vi "SendMessage.vi"(0 "reference in":refnum<class "Colleague.lvclass">, 4 "Receiver":string, 5 "error in (no error)":errorcluster, 8 "Message":string) -> (14 "reference out":refnum<class "Colleague.lvclass">, 19 "error out":errorcluster)   [LabVIEW 2013, in "Colleague.lvclass"]
uses:
  Colleague.lvclass
  Mediator_class/Mediator.lvclass
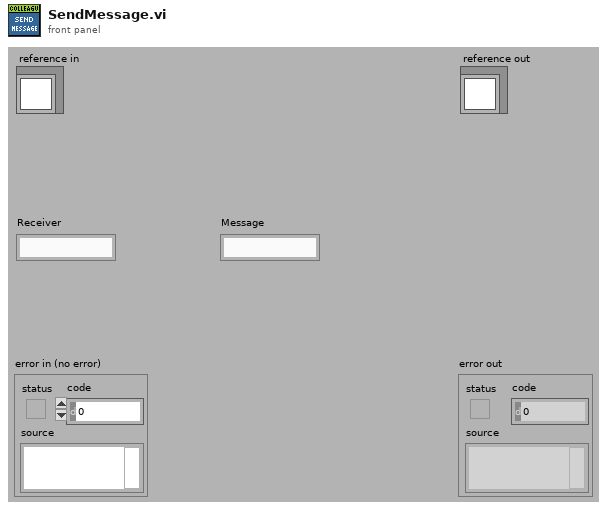
[diagram p1: front panel]
types:
  T1 = typedef "Colleague.lvclass/ObjectAttributes.ctl" = cluster{"Name":string, "Mediator.lvclass":refnum<class "Mediator.lvclass">}
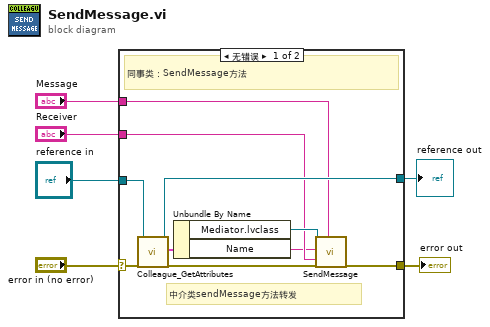
[diagram p0: block diagram]
diagram:
  n1 = case shown="无错误" "error in (no error)" {
    selector: "error in (no error)" -> [w16 w18]
    tunnel: [w7 w18] -> w5
    tunnel: [w15 w17] -> w3
    tunnel: "reference in" -> [w13 w17]
    tunnel: "Receiver" -> [w11 _]
    tunnel: "Message" -> [w10 _]
    frame No Error {
      # "中介类sendMessage方法转发"
      # "同事类：SendMessage方法"
      n2 = call "Colleague_GetAttributes.vi"("reference in"=w13, "error in (no error)"=w16) -> ("reference out"=w15:refnum<class "Colleague.lvclass">, "attributes"=w14:T1, "error out"=w8:errorcluster)  [unwired: 14 in, 1 out]
      n3 = Unbundle By Name(w14) -> ("Mediator.lvclass"=w12:refnum<class "Mediator.lvclass">, "Name"=w9:string)
      n4 = call-dynamic "SendMessage.vi"("reference in"=w12, "Sender"=w9, "Receiver"=w11, "error in (no error)"=w8, "Message"=w10) -> ("error out"=w7:errorcluster)  [unwired: 13 in, 1 out]
    }
    frame Error {
    }
  }
  "error out" <- w5
  "reference out" <- w3
